vi "Model Network Steam.vi"(8 "error in (no error)":errorcluster, 11 "Model in":refnum<class "Model.lvclass">) -> (0 "error out":errorcluster)   [LabVIEW 2021, in "Model.lvlib" / "Model.lvclass"]
uses:
  Model.lvclass
  <userlib>/John_Lib/Network_Streams_Connection/NetworkCommand--Cluster.ctl
  Model.lvclass/Model.ctl
  ebfee82e-1d41-4e87-aba7-8c7096a207ef.vi
  cbdd33bf-e0af-482d-9349-bbda270fe613.vi
  <userlib>/John_Lib/AMC_FW/Read Next Message.vi
  <userlib>/John_Lib/AMC_FW/Parse State Queue__JKI.vi
  <userlib>/John_Lib/AMC_FW/Send Local Message.vi
  <userlib>/John_Lib/AMC_FW/Read Termination Message.vi
  <userlib>/John_Lib/AMC_FW/Create Single Message.vi
  <userlib>/John_Lib/AMC_FW/Update Message Routing Info.vi
  <userlib>/John_Lib/AMC_FW/Globals.vi
  <vilib>/Utility/error.llb/Trim Whitespace.vi
  <userlib>/John_Lib/AMC_FW/String to Array.vi
  <userlib>/John_Lib/AMC_FW/Send Message.vi
  <userlib>/John_Lib/AMC_FW/AMC_FW.lvlib
  <userlib>/John_Lib/Network_Streams_Connection/NetworkConnection.lvclass
panel:
  in  "Timeout(ms)":i32=1000
  out "Messages":T1[](array[typedef])
  out "Timed Out?":bool
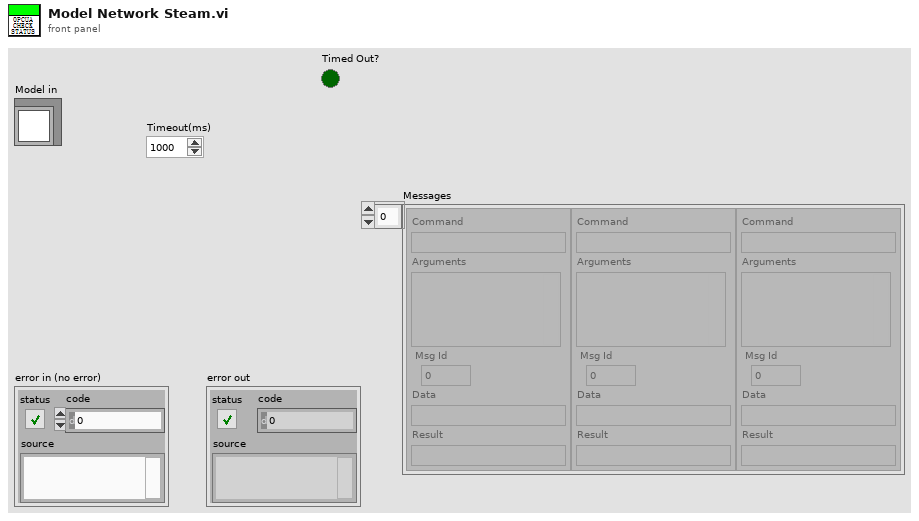
[diagram p1: front panel]
types:
  T1 = typedef "JKI_Network_Streams.lvlib/NetworkConnection.lvclass/NetworkCommand--Cluster.ctl" = cluster{"Command":string, "Arguments":variant, " Msg Id":i32, "Data":string, "Result":string}
  T2 = typedef "AMC_FW.lvlib/Queue.ctl" = cluster{"Q":T3, "Name":string}
  T3 = typedef "AMC_FW.lvlib/Message Queue.ctl" = refnum<queue>
  T4 = typedef "Model.lvlib/Model.lvclass/DVR.ctl" = cluster{"JKI_Network_Streams":refnum<class "NetworkConnection.lvclass">, "AMC Q":T5}
  T5 = typedef "Model.lvlib/Model.lvclass/AMC Q.ctl" = cluster{"Main":T2, "OPCUA":T2, "NetworkSteam":T2}
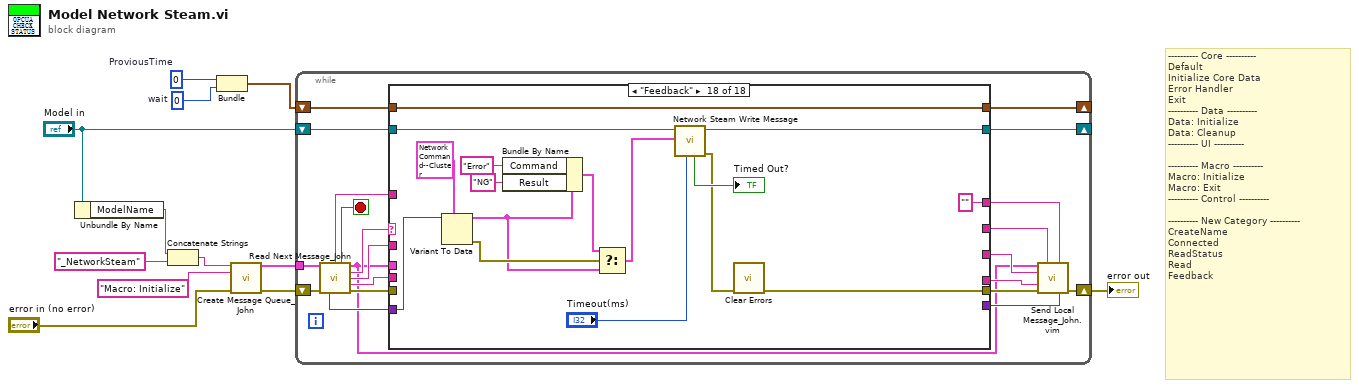
[diagram p0: block diagram]
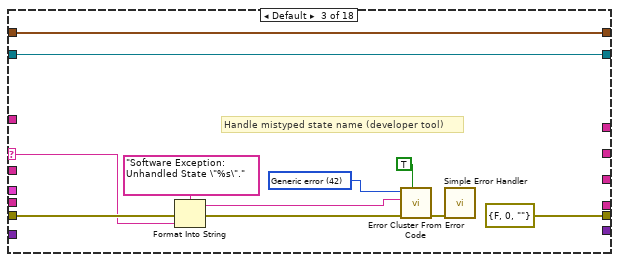
[diagram p4: hidden frame]
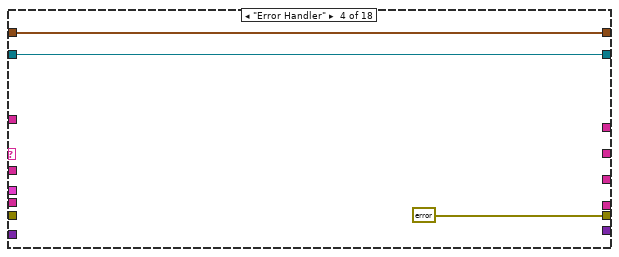
[diagram p5: hidden frame]
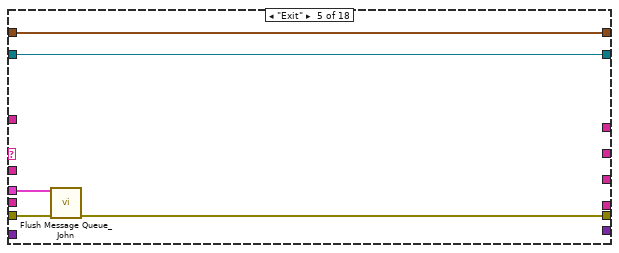
[diagram p6: hidden frame]
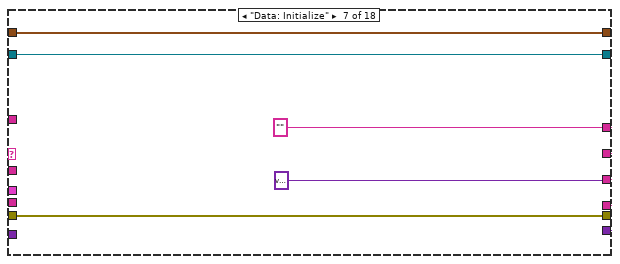
[diagram p8: hidden frame]
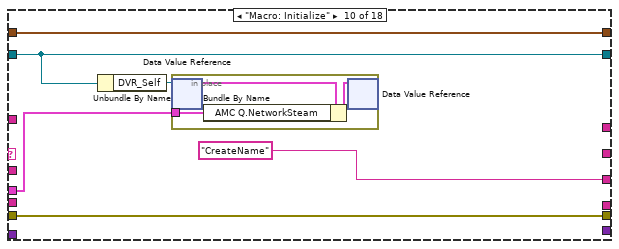
[diagram p11: hidden frame]
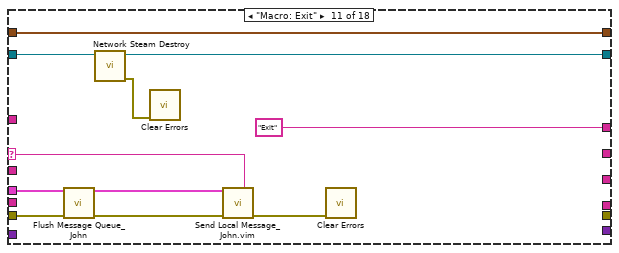
[diagram p12: hidden frame]
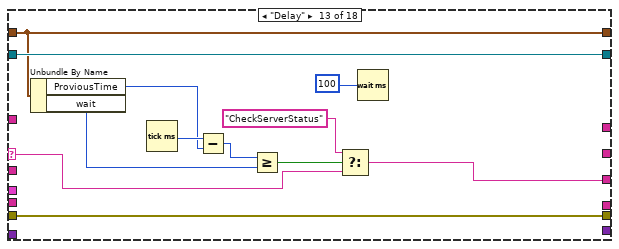
[diagram p14: hidden frame]
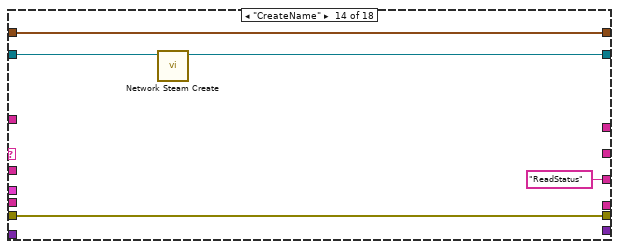
[diagram p15: hidden frame]
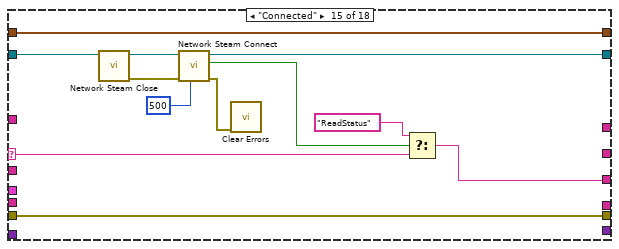
[diagram p16: hidden frame]
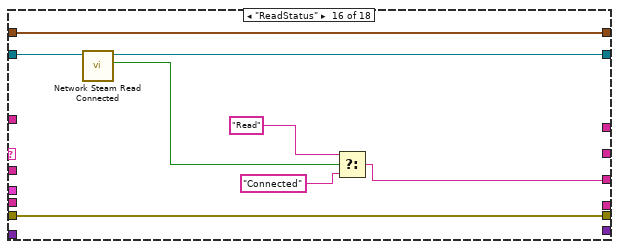
[diagram p17: hidden frame]
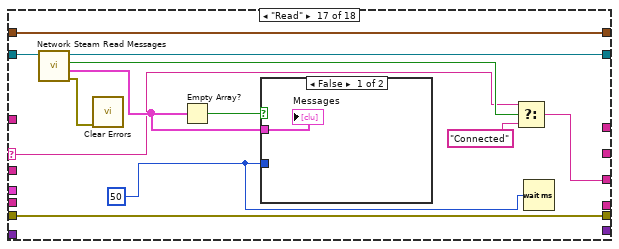
[diagram p18: hidden frame]
diagram:
  w4 = u32 0  # wait
  w11 = u32 0  # ProviousTime
  # "---------- Core ----------\nDefault\nInitialize Core Data\nError Handler\nExit\n---------- Data ----------\nData: Initialize\nData: Cleanup\n---------- UI ----------\n\n---------- Macro ----------\nMacro: Initialize\nMacro: Exit\n---------- Control ----------\n\n---------- New Category ----------\nCreateName\nConnected\nReadStatus\nRead\nFeedback"
  n1 = Unbundle By Name("Model in") -> ("ModelName"=w5:string)
  n2 = Concatenate Strings(w5, "_NetworkSteam" ("string")) -> (w1:string)
  n3 = Bundle("ProviousTime"=w11, "wait"=w4) -> (w10:cluster{"ProviousTime":u32, "wait":u32})  [unwired: 1 in]
  n4 = call <userlib>:"Create Message Queue_John.vi"("message queue name"=w1, "initial message names"="Macro: Initialize", "error in"="error in (no error)") -> ("message queue out"=w8:T2, "error out"=w7:errorcluster)  [unwired: 11 in]
  n5 = while {
    shift-right: [w24] -> w12
    shift-left: w7 -> [w32]
    shift-right: [w33] -> _
    shift-left: "Model in" -> [w26]
    tunnel: w8 -> [w29]
    shift-right: [w14] -> _
    shift-left: w10 -> [w15]
    stop <- w16 stop-if-true
    n6 = call <userlib>:"Read Next Message_John.vi"("Queue In"=w29, "error in"=w32) -> ("Previous State + Arguments"=w25:string, "exit process?"=w16:bool, "Queue Out"=w13:T2, "Current State"=w30:string, "Arguments"=w28:string, "message value"=w27:string, "variant"=w17:variant, "error out"=w31:errorcluster)  [unwired: 4 in, 2 out]
    n7 = case shown="\"Feedback\"" w30 {
      selector: w30 -> [_ _ w45 _ _ _ _ _ _ _ w82 _ w99 _ w115 _ w136 _]
      tunnel: w13 -> [_ _ _ _ w56 _ _ _ _ w73 w92 _ _ _ _ _ _ _]
      tunnel: w27 -> [_ _ _ _ _ _ _ _ _ _ _ _ _ _ _ _ _ _]
      tunnel: [w35 w39 errorcluster {"status"=FALSE, "code"=0, "source"=""} ("error out") errorcluster {"status"=FALSE, "code"=0, "source"=""} ("error out") w57 w60 w66 w68 w71 w78 _ w95 w107 w112 w124 w132 w144 w146] -> w23
      tunnel: w31 -> [w35 w39 w46 _ w58 w60 w66 w68 w71 w78 w91 w95 w107 w112 w124 w132 w144 _]
      tunnel: w26 -> [w36 w38 w42 w53 w55 w61 w64 w69 w72 w74 w87 w94 w106 w109 w118 w129 w142 w159]
      tunnel: [w36 w38 w42 w53 w55 w61 w64 w69 w72 w74 w88 w94 w106 w110 w119 w130 w141 w160] -> w33
      tunnel: w28 -> [_ _ _ _ _ _ _ _ _ _ _ _ _ _ _ _ _ _]
      tunnel: w25 -> [_ _ _ _ _ _ _ _ _ _ _ _ _ _ _ _ _ _]
      tunnel: [_ _ _ _ _ _ w65 _ _ _ _ _ _ _ _ _ _ _] -> w22
      tunnel: [_ _ _ _ _ _ w65 _ _ _ "Exit" _ _ _ _ _ _ "" ("Elements in Front")] -> w21
      tunnel: [_ _ _ _ _ _ w65 _ _ "CreateName" _ _ w98 "ReadStatus" ("initial message names") w114 w125 w135 _] -> w20
      tunnel: [_ _ _ _ _ _ w65 _ _ _ _ _ _ _ _ _ _ _] -> w19
      tunnel: [_ _ _ _ _ _ variant ("variant") _ _ _ _ _ _ _ _ _ _ _] -> w18
      tunnel: w17 -> [_ _ _ _ _ _ _ _ _ _ _ _ _ _ _ _ _ w156]
      tunnel: w15 -> [w34 w37 w40 w51 w54 w59 w62 w67 w70 w76 w89 w93 w105 w111 w123 w131 w143 w161]
      tunnel: [w34 w37 w40 w51 w54 w59 w62 w67 w70 w76 w89 w93 w105 w111 w123 w131 w143 w161] -> w14
      frame "", "Idle" {
      }
      frame "---------- Core ----------" {
      }
      frame Default {
        w48 = 42 items=["No error", "Argument error", "Memory is full", "Out of zone", "End of file", "File already open", "Generic file I/O error", "File not found", "File permission error", "Disk is full", "Duplicate path", "Too many files open", "System feature not enabled", "Resource file not found", "Cannot add resource", "Resource not found", "Image not found", "Image memory error", "Pen does not exist", "Config type invalid", "Config token not found", "Config parse error", "Config memory error", "Bad external code format", "Bad external code offset", "External code not present", "Null window", "Destroy window error", "Null menu", "Print aborted", "Bad print record", "Print driver error", "Windows error during printing", "Memory error during printing", "Print dialog error", "Generic print error", "Invalid device refnum", "Device not found", "Device parameter error", "Device unit error", "Cannot open device", "Device call aborted", "Generic error", "Cancelled by user", "Object ID too low", "Object ID too high", "Object not in heap", "Unknown heap", "Unknown object (invalid DefProc)", "Unknown object (DefProc not in table)", "Message out of range", "Invalid (null) method", "Unknown message", "Manager call not supported", "Bad address", "Network operation in progress", "Network operation timed out", "Connection is busy", "Network attribute not supported", "Network error", "Address in use", "System out of memory", "Connection aborted", "Connection refused", "Not connected", "Already connected", "Connection closed", "Initialization error (interapplication manager)", "Bad occurrence", "Wait on unbound occurrence handler", "Occurrence queue overflow", "Datalog type conflict", "Unused", "Unrecognized type (interapplication manager)", "Memory corrupt", "Failed to make temporary DLL", "Old CIN version", "Drag socket not found", "Failed to load drop-object", "Failed to register OLE object", "Failed to release OLE object", "Format specifier type mismatch", "Unknown format specifier", "Too few format specifiers", "Too many format specifiers", "Scan failed", "Newer CIN version", "Error converting to variant", "Runtime menu error", "Password tampered", "Variant attribute not found", "Incompatible variant data type", "Event data is not available", "Event Store is not present", "Occurrence is not found", "Event Queue is not created", "Event info is not available", "Refnum passed is NULL", "Error retrieving Class GUID", "Error retrieving CoClass GUID", "Error retrieving TypeLib GUID.", "Bad built application magic bytes.", "Specific driver is different from the specific driver associated with the Logical Name.", "There is no session opened to the class driver.", "Max Error", "MAX - Error with config objects", "MAX - Error loading configuration", "MAX - Group not supported"]
        # "Handle mistyped state name (developer tool)"
        n8 = Format Into String(format string="Software Exception: Unhandled State \"%s\"." ("message"), error in=w46, w45) -> (resulting string=w41:string, error out=w49:errorcluster)  [unwired: 1 in]
        n9 = call <vilib>:"Error Cluster From Error Code.vi"("show call chain? (False)"=TRUE, "error in (no error)"=w49, "error message (\"\")"=w41, "error code (0)"=w48) -> ("error out"=w44:errorcluster)  [unwired: 5 in]
        n10 = call <vilib>:"Simple Error Handler.vi"("error in (no error)"=w44) -> ()  [unwired: 4 in, 5 out]
      }
      frame "Error Handler" {
      }
      frame "Exit" {
        n11 = call <userlib>:"Flush Message Queue_John.vi"("Queue In"=w56, "error in"=w58) -> ("error out"=w57:errorcluster)  [unwired: 11 in, 2 out]
      }
      frame "---------- Data ----------" {
      }
      frame "Data: Initialize" {
        w65 = "" ("Elements in Front")
      }
      frame "---------- UI ----------" {
      }
      frame "---------- Macro ----------" {
      }
      frame "Macro: Initialize" {
        n12 = Unbundle By Name(w74) -> ("DVR_Self"=w75:refnum<data-value>)
        n13 = in-place {
          in-place-border: w73 -> [w79]
          n14 = in-place-dvr #1(w75) -> (w81:T4)  [unwired: 1 out]
          n15 = Bundle By Name(cluster=w81, "AMC Q.NetworkSteam"=w79) -> (w80:T4)
          n16 = in-place-dvr #1(w80) -> ()  [unwired: 2 out]
        }
      }
      frame "Macro: Exit" {
        n17 = call <userlib>:"Flush Message Queue_John.vi"("Queue In"=w92, "error in"=w91) -> ("Queue Out"=w84:T2, "error out"=w85:errorcluster)  [unwired: 11 in, 1 out]
        n18 = call "Network Steam Destroy.vi"("Model in"=w87) -> ("error out"=w86:errorcluster, "Model out"=w88:refnum<class "Model.lvclass">)  [unwired: 9 in]
        n19 = call <vilib>:"Clear Errors.vi"("error in (no error)"=w86) -> ()  [unwired: 5 in, 2 out]
        n20 = call "Send Local Message_John.vim"("Queue In"=w84, "Elements in Front"=w82, "error in"=w85) -> ("error out"=w83:errorcluster)  [unwired: 10 in, 2 out]
        n21 = call <vilib>:"Clear Errors.vi"("error in (no error)"=w83) -> ()  [unwired: 5 in, 2 out]
      }
      frame "---------- Control ----------" {
      }
      frame "Delay" {
        n22 = Unbundle By Name(w105) -> ("ProviousTime"=w103:u32, "wait"=w96:u32)
        n23 = Tick Count (ms)() -> (millisecond timer value=w104:u32)
        n24 = Subtract(x=w104, y=w103) -> (x-y=w102:u32)
        n25 = Greater Or Equal?(x=w102, y=w96) -> (x >= y?=w101:bool)
        n26 = Select(t="CheckServerStatus" ("Previous State + Arguments"), s=w101, f=w99) -> (s? t:f=w98:string)
        n27 = Wait (ms)(milliseconds to wait=u32 100) -> ()  [unwired: 1 out]
      }
      frame "CreateName" {
        n28 = call "Network Steam Create.vi"("Model in"=w109) -> ("Model out"=w110:refnum<class "Model.lvclass">)  [unwired: 9 in, 1 out]
      }
      frame "Connected" {
        n29 = call "Network Steam Close.vi"("Model in"=w118) -> ("error out"=w121:errorcluster, "Model out"=w122:refnum<class "Model.lvclass">)  [unwired: 9 in]
        n30 = call "Network Steam Connect.vi"("Timeout(ms)"=500, "error in (no error)"=w121, "Model in"=w122) -> ("error out"=w113:errorcluster, "Connected?"=w117:bool, "Model out"=w119:refnum<class "Model.lvclass">)  [unwired: 6 in]
        n31 = call <vilib>:"Clear Errors.vi"("error in (no error)"=w113) -> ()  [unwired: 5 in, 2 out]
        n32 = Select(t="ReadStatus" ("initial message names"), s=w117, f=w115) -> (s? t:f=w114:string)
      }
      frame "ReadStatus" {
        n33 = call "Network Steam Read Connected.vi"("Model in"=w129) -> ("Connected?"=w128:bool, "Model out"=w130:refnum<class "Model.lvclass">)  [unwired: 8 in, 1 out]
        n34 = Select(t="Read", s=w128, f="Connected" ("initial message names")) -> (s? t:f=w125:string)
      }
      frame "Read" {
        w133 = u32 50 ("milliseconds to wait")
        n35 = call "Network Steam Read Messages.vi"("Model in"=w142) -> ("error out"=w140:errorcluster, "Messages"=w138:T1[], "StillConnected?"=w137:bool, "Model out"=w141:refnum<class "Model.lvclass">)  [unwired: 6 in, 1 out]
        n36 = call <vilib>:"Clear Errors.vi"("error in (no error)"=w140) -> ()  [unwired: 5 in, 2 out]
        n37 = Empty Array?(array=w138) -> (empty?=w139:bool)
        n38 = case shown="False" w139 {
          tunnel: w138 -> [w145 _]
          tunnel: w133 -> [_ _]
          frame False {
            "Messages" <- w145
          }
          frame True {
          }
        }
        n39 = Select(t=w136, s=w137, f="Connected") -> (s? t:f=w135:string)
        n40 = Wait (ms)(milliseconds to wait=w133) -> ()  [unwired: 1 out]
      }
      frame "Feedback" {
        n41 = Variant To Data(type=T1 {"Command"="", "Arguments"=variant, " Msg Id"=-1, "Data"="", "Result"=""} ("Message"), Variant=w156) -> (data=w152:T1, error out=w154:errorcluster)  [unwired: 1 in]
        n42 = Bundle By Name(cluster=w152, "Command"="Error", "Result"="NG") -> (w151:T1)
        n43 = Select(t=w151, s=w154, f=w152) -> (s? t:f=w153:T1)
        n44 = call "Network Steam Write Message.vi"("Timeout(ms)"="Timeout(ms)", "Message"=w153, "Model in"=w159) -> ("error out"=w148:errorcluster, "Model out"=w160:refnum<class "Model.lvclass">, "Timed Out?"=→"Timed Out?":bool)  [unwired: 5 in, 1 out]
        n45 = call <vilib>:"Clear Errors.vi"("error in (no error)"=w148) -> ("error out"=w146:errorcluster)  [unwired: 5 in, 1 out]
      }
    }
    n46 = call "Send Local Message_John.vim"("Queue In"=w13, "receiver process (\"\" - local)"=w22, "Elements in Front"=w21, "Elements at Back"=w20, "message value"=w19, "error in"=w23, "variant"=w18) -> ("error out"=w24:errorcluster)  [unwired: 6 in, 2 out]
  }
  "error out" <- w12
